vi "ABB Test Cooling curve.vi"(10 "Measure":enum16{"Full Load", "Partial Load", "No Load"}(ring), 11 "Heat run Type":enum16{"Full Load", "Partial- & No-Load"}(ring)) -> ()   [LabVIEW 2017]
uses:
  ABB global.vi
panel:
  in  "Slip Ring Temperatures (° C)":cluster{"K":dbl, "L":dbl, "M ":dbl}
  out "Selection":T1 {"Rotor dT" format="%#.2g"; "Rotor R" format="%#.6g"; "Stator dT" format="%#.2g"; "Stator R" format="%#.6g"}
  in  "Use":bool
  out "Rotor Fitted Zero time  R":dbl format="%.4f"
  out "Type of Run":string
  in  "Stop":bool
  out "Elapsed time (secs)":dbl format="%#.1f"
  in  "Start":bool
  in  "Enter Rotor Res.":dbl
  in  "Enter Stator Res.":dbl
  in  "Select Resistance":T2(ring)
  out "Motor Type":string
  out "Cooling in Temp (°C)":dbl
  out "error":dbl
  in  "y":dbl step=0.01
  out "Stator Fitted Zero time  R":dbl format="%.4f"
  out "Selected Entries 2":string[](array[string])
  out "Cold resistance":T3 {"Temperature(°C)" format="%#.2g"}
  in  "Rotor Cooling Curve Data":string[][](table)
  out "Rotor":cluster{dbl[], dbl[]}[](graph)
  out "Rotor Readings":string[][](table)
  in  "Stator Cooling Curve Data":string[][](table)
  out "Stator":cluster{dbl[], dbl[]}[](graph)
  out "Stator Readings":string[][](table)
  out "Serial number":string
  out "W.O number":string
  out "Timedate":string
  in  "Exit":bool
  # "?"
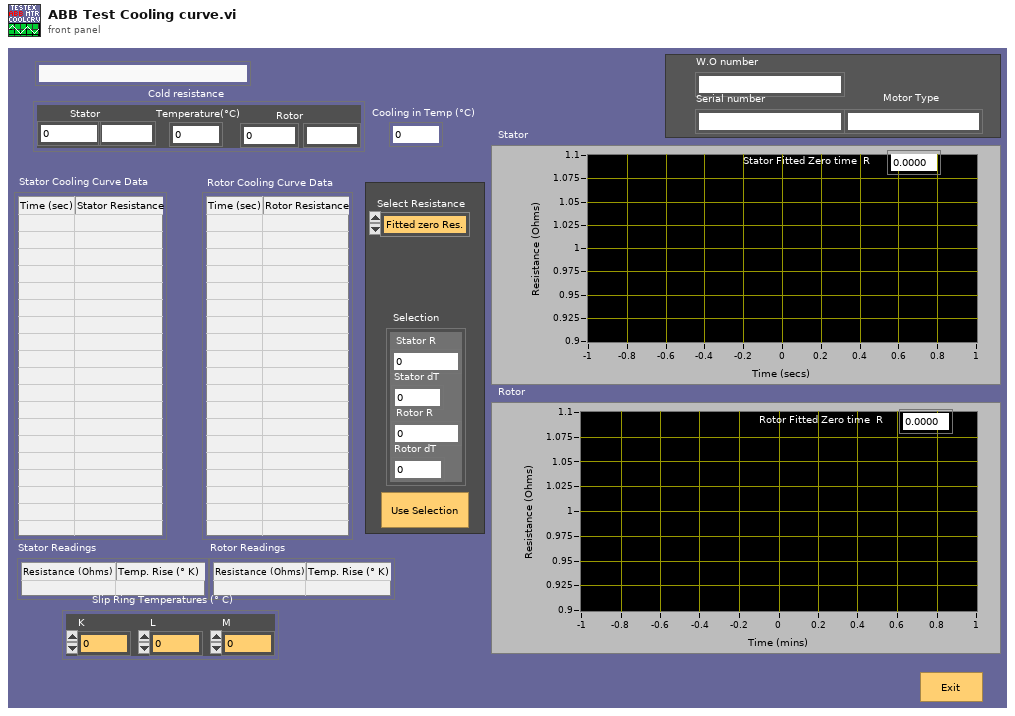
[diagram p1: front panel]
types:
  T1 = cluster{"Stator R":dbl, "Stator dT":dbl, "Rotor R":dbl, "Rotor dT":dbl}
  T2 = enum16{"Fitted zero Res.", "Selected Res.", "Entered Res."}
  T3 = cluster{"Stator":dbl, "Rotor":dbl, "Stator Units":string, "Rotor Units":string, "Temperature(°C)":dbl}
  T4 = cluster{"Stator R":dbl, "Stator dT":dbl, "Rotor R":dbl, "Rotor dT":dbl, "Stator Cooling curve":dbl[][], "Rotor Cooling curve":dbl[][], "Select Resistance":enum16{"Fitted zero Res.", "Selected Res.", "Entered Res."}}[]
  T5 = cluster{"Stator R":dbl, "Stator dT":dbl, "Rotor R":dbl, "Rotor dT":dbl, "Stator Cooling curve":dbl[][], "Rotor Cooling curve":dbl[][], "Select Resistance":enum16{"Fitted zero Res.", "Selected Res.", "Entered Res."}}
  T6 = cluster{"Simulate Norma":bool, "Norma 5000 Address":u8, "WebDaq IP Address":string, "Simulate cDAQ":bool}
  T7 = typedef "LVRowAndColumnTypeDef.ctl" = cluster{"Row":i32, "Column":i32}
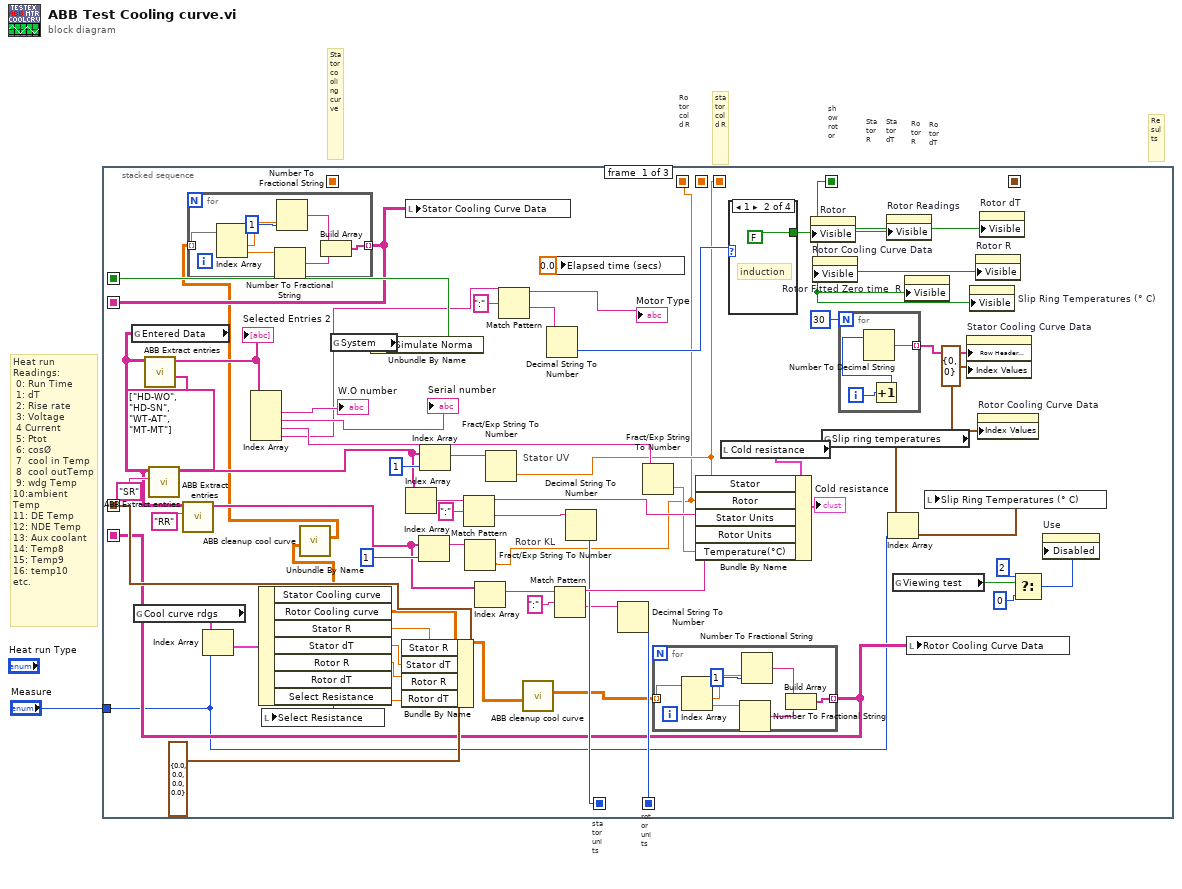
[diagram p0: block diagram]
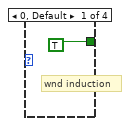
[diagram p2: hidden frame]
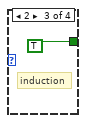
[diagram p3: hidden frame]
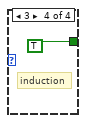
[diagram p4: hidden frame]
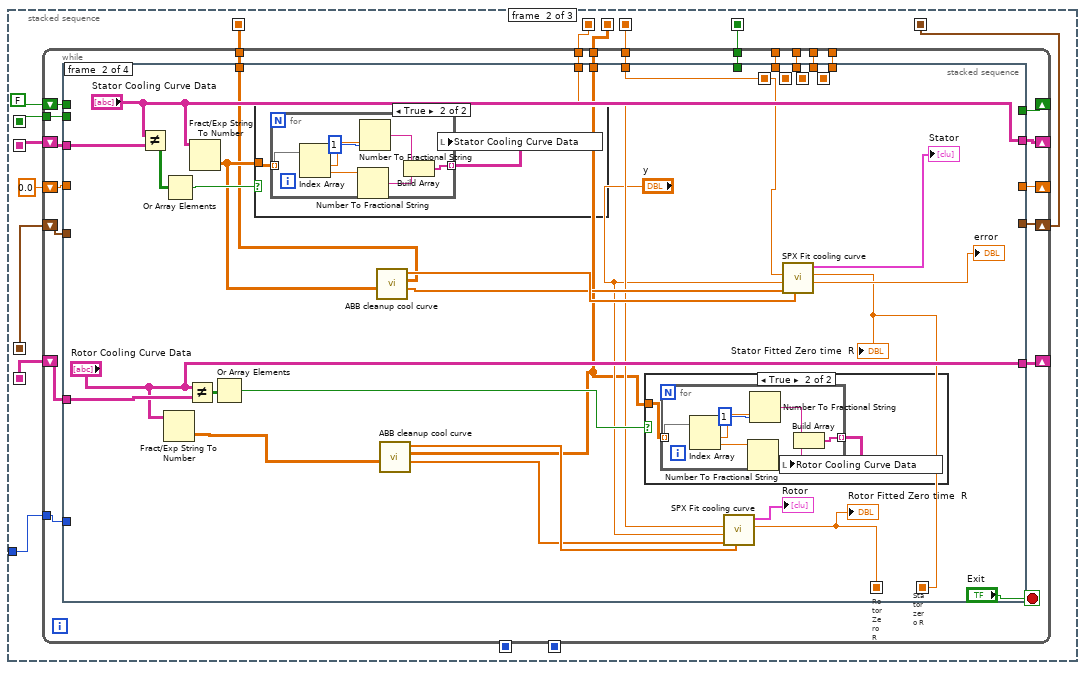
[diagram p5: hidden frame]
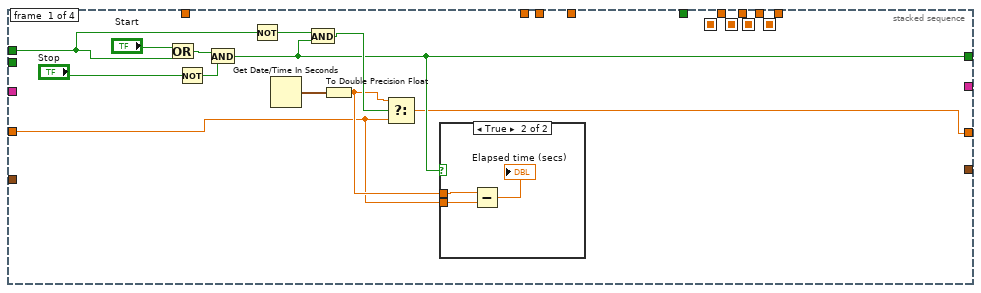
[diagram p6: hidden frame]
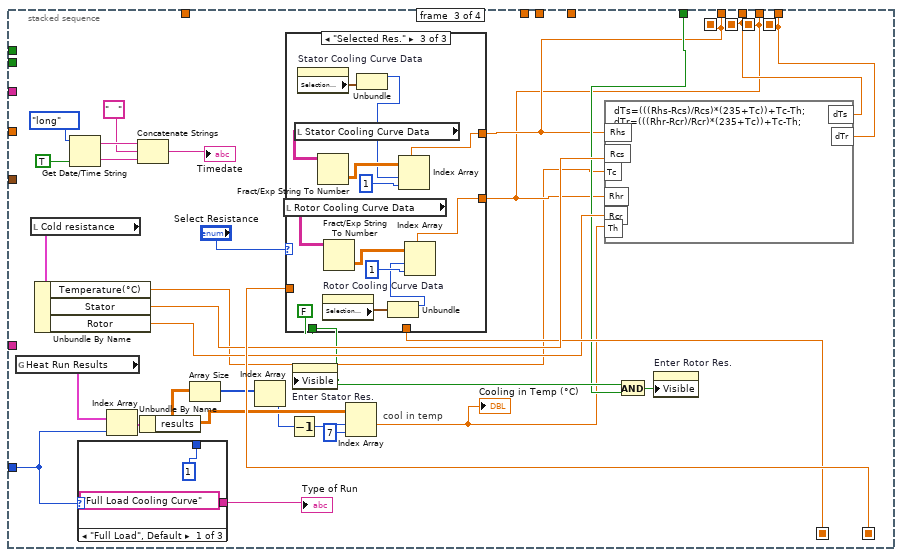
[diagram p10: hidden frame]
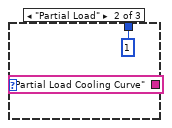
[diagram p11: hidden frame]
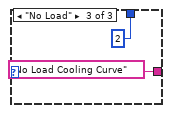
[diagram p12: hidden frame]
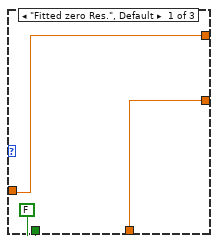
[diagram p13: hidden frame]
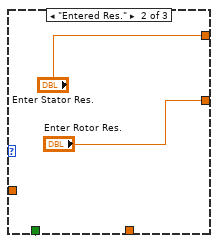
[diagram p14: hidden frame]
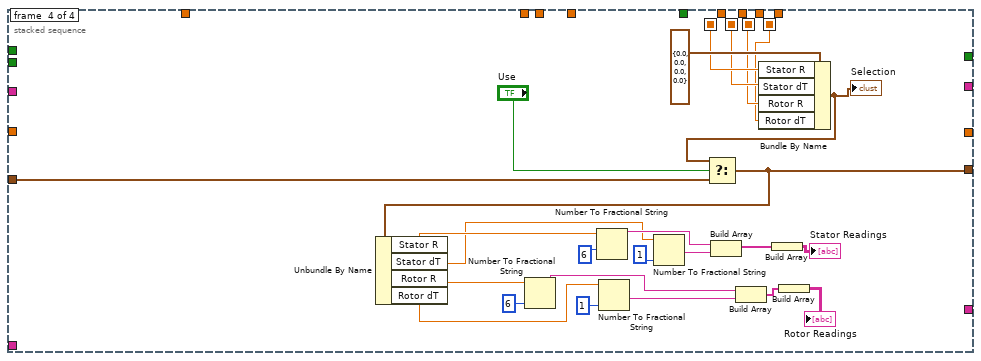
[diagram p15: hidden frame]
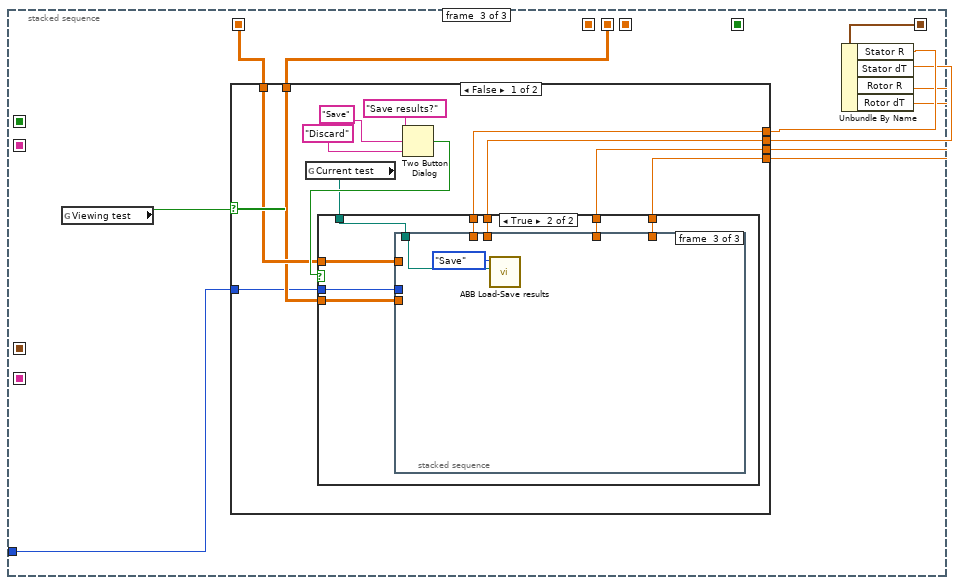
[diagram p16: hidden frame]
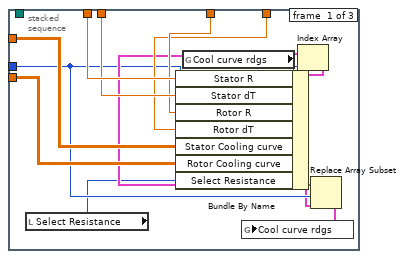
[diagram p18: hidden frame]
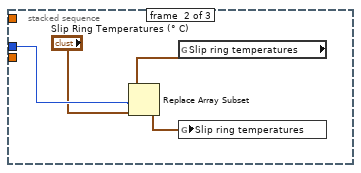
[diagram p19: hidden frame]
diagram:
  # "StatordT"
  # "RotordT"
  # "Rotor R"
  # "Stator R"
  # "show rotor"
  # "Rotor cold R"
  # "Heat run Readings:\n 0: Run Time\n 1: dT\n 2: Rise rate\n 3: Voltage\n 4 Current\n 5: Ptot\n 6: cosØ\n 7  cool in Temp\n 8  cool outTemp\n 9: wdg Temp\n10:ambient Temp\n11: DE Temp\n12: NDE Temp\n13: Aux coolant\n14: Temp8\n15: Temp9\n16: temp10\netc."
  # "rotor units"
  # "stator units"
  # "Stator cooling curve"
  # "stator cold R"
  # "Results"
  n1 = stacked-sequence {
    seq-local: [w63 _ _] -> [_ w98 _]
    seq-local: [w10 _ _] -> [_ w97 _]
    seq-local: [_ w96 _] -> [_ _ w265]
    seq-local: [_ w95 _] -> [_ _ w264]
    seq-local: [w11 _ _] -> [_ w94 _]
    seq-local: [w19 _ _] -> [_ w93 _]
    seq-local: [w32 _ _] -> [_ _ _]
    seq-local: [w30 _ _] -> [_ _ _]
    seq-local: [w18 _ _] -> [_ w92 _]
    seq-local: [w8 _ _] -> [_ w91 _]
    seq-local: [w20 _ _] -> [_ w87 _]
    seq-local: [_ w86 _] -> [_ _ w262]
    tunnel: "Measure" -> [w2 w88 w263]
    frame #0 {
      w5 = cluster{"Row":i32, "Column":i32} {"Row"=0, "Column"=0} ("Edit Position")
      # "Rotor KL"
      # "Stator UV"
      n2 = global read "ABB global.vi" "Entered Data"() -> (w56:string[][])
      n3 = global read "ABB global.vi" "Cool curve rdgs"() -> (w27:T4)
      n4 = call "ABB Extract entries.vi"("Entry IDs"=string[] ["HD-WO", "HD-SN", "WT-AT", "MT-MT"], "Entry table in"=w56) -> ("Selected Entries"=w39:string[])  [unwired: 9 in]
      "Selected Entries 2" <- w39
      n5 = call "ABB Extract entries.vi"("Entry ID"="SR", "Entry table in"=w56) -> ("Selected Entries"=w50:string[])  [unwired: 9 in]
      n6 = call "ABB Extract entries.vi"("Entry ID"="RR", "Entry table in"=w56) -> ("Selected Entries"=w43:string[])  [unwired: 9 in]
      n7 = Index Array(array=w27, index=w2) -> (element=w26:T5)
      n8 = Index Array(array=w39) -> (element #1=→"W.O number":string, element #2=→"Serial number":string, element #3=w40:string, element #4=w35:string)  [unwired: 4 in]
      n9 = Unbundle By Name(w26) -> ("Stator Cooling curve"=w12:dbl[][], "Rotor Cooling curve"=w9:dbl[][], "Stator R"=w25:dbl, "Stator dT"=w24:dbl, "Rotor R"=w23:dbl, "Rotor dT"=w22:dbl, "Select Resistance"=w13:T2)
      n10 = local write "Select Resistance"(w13) -> ()
      n11 = call "ABB cleanup cool curve.vi"("cool curve in"=w12) -> ("Cool curve out"=w7:dbl[][])  [unwired: 8 in, 2 out]
      n12 = for {
        tunnel: w7 -> [w78] mode=indexing
        tunnel: [w74] -> w11 mode=indexing
        n13 = Index Array(array=w78) -> (element #1=w76:dbl, element #2=w75:dbl)  [unwired: 2 in]
        n14 = Number To Fractional String(number=w75) -> (F-format string=w73:string)  [unwired: 3 in]
        n15 = Number To Fractional String(number=w76, precision (6)=i16 1) -> (F-format string=w72:string)  [unwired: 2 in]
        n16 = Build Array(w72, w73) -> (w74:string[])
      }
      n17 = global read "ABB global.vi" "System"() -> (w64:T6)
      n18 = Unbundle By Name(w64) -> ("Simulate Norma"=w63:bool)
      n19 = Bundle By Name(cluster=T1 {"Stator R"=0.0, "Stator dT"=0.0, "Rotor R"=0.0, "Rotor dT"=0.0} ("Selection"), "Stator R"=w25, "Stator dT"=w24, "Rotor R"=w23, "Rotor dT"=w22) -> (w20:T1)
      n20 = local write "Stator Cooling Curve Data"(w11) -> ()
      n21 = Index Array(array=w50) -> (element=w49:string)  [unwired: 1 in]
      n22 = Index Array(array=w43, index=1) -> (element=w45:string)
      n23 = Index Array(array=w50, index=1) -> (element=w53:string)
      n24 = Match Pattern(string=w49, regular expression=":") -> (before substring=w42:string, after substring=w33:string)  [unwired: 1 in, 2 out]
      n25 = Fract/Exp String To Number(string=w45) -> (number=w18:dbl)  [unwired: 3 in, 1 out]
      n26 = Index Array(array=w43) -> (element=w46:string)  [unwired: 1 in]
      n27 = Fract/Exp String To Number(string=w53) -> (number=w19:dbl)  [unwired: 3 in, 1 out]
      n28 = Match Pattern(string=w35, regular expression=":") -> (before substring=→"Motor Type":string, after substring=w37:string)  [unwired: 1 in, 2 out]
      n29 = call "ABB cleanup cool curve.vi"("cool curve in"=w9) -> ("Cool curve out"=w6:dbl[][])  [unwired: 8 in, 2 out]
      n30 = Decimal String To Number(string=w37) -> (number=w34:i32)  [unwired: 2 in, 1 out]
      n31 = local write "Elapsed time (secs)"(0.0 ("Elapsed time (secs)")) -> ()
      n32 = Match Pattern(string=w46, regular expression=":") -> (before substring=w41:string, after substring=w31:string)  [unwired: 1 in, 2 out]
      n33 = Decimal String To Number(string=w33) -> (number=w32:i32)  [unwired: 2 in, 1 out]
      n34 = Decimal String To Number(string=w31) -> (number=w30:i32)  [unwired: 2 in, 1 out]
      n35 = Fract/Exp String To Number(string=w40) -> (number=w29:dbl)  [unwired: 3 in, 1 out]
      n36 = for {
        tunnel: w6 -> [w71] mode=indexing
        tunnel: [w67] -> w10 mode=indexing
        n37 = Index Array(array=w71) -> (element #1=w69:dbl, element #2=w68:dbl)  [unwired: 2 in]
        n38 = Number To Fractional String(number=w68) -> (F-format string=w66:string)  [unwired: 3 in]
        n39 = Number To Fractional String(number=w69, precision (6)=i16 1) -> (F-format string=w65:string)  [unwired: 2 in]
        n40 = Build Array(w65, w66) -> (w67:string[])
      }
      n41 = local read "Cold resistance"() -> (w52:T3)
      n42 = Bundle By Name(cluster=w52, "Stator"=w19, "Rotor"=w18, "Stator Units"=w42, "Rotor Units"=w41, "Temperature(°C)"=w29) -> (→"Cold resistance":T3)
      n43 = case shown="1" w34 {
        tunnel: [TRUE FALSE TRUE TRUE] -> w8
        frame 0, Default {
          # "wnd induction"
        }
        frame 1 {
          # "induction"
        }
        frame 2 {
          # "induction"
        }
        frame 3 {
          # "induction"
        }
      }
      n44 = property on="Rotor" class="XYGraph (strict)"("Visible"=w8) -> ()  [unwired: 2 in, 2 out]
      n45 = property on="Rotor Cooling Curve Data" class="Tbl (strict)"("Visible"=w8) -> ()  [unwired: 2 in, 2 out]
      n46 = global read "ABB global.vi" "Slip ring temperatures"() -> (w4:cluster{"K":dbl, "L":dbl, "M ":dbl}[])
      n47 = for {
        N: 30 -> [_]
        tunnel: [w83] -> w61 mode=indexing
        i -> [w85]
        n48 = Increment(x=w85) -> (x+1=w84:i32)
        n49 = Number To Decimal String(number=w84) -> (decimal integer string=w83:string)  [unwired: 1 in]
      }
      n50 = property on="Rotor Readings" class="Tbl (strict)"("Visible"=w8) -> ()  [unwired: 2 in, 2 out]
      n51 = Index Array(array=w4, index=w2) -> (element=w3:cluster{"K":dbl, "L":dbl, "M ":dbl})
      n52 = global read "ABB global.vi" "Viewing test"() -> (w17:bool)
      n53 = property on="Rotor Fitted Zero time  R" class="DigNum (strict)"("Visible"=w8) -> ()  [unwired: 2 in, 2 out]
      n54 = local write "Rotor Cooling Curve Data"(w10) -> ()
      n55 = local write "Slip Ring Temperatures (° C)"(w3) -> ()
      n56 = property on="Stator Cooling Curve Data" class="Tbl (strict)"("Row Header Strings[]"=w61, "Index Values"=w5) -> ()  [unwired: 2 in, 2 out]
      n57 = property on="Slip Ring Temperatures (° C)" class="Clust (strict)"("Visible"=w8) -> ()  [unwired: 2 in, 2 out]
      n58 = property on="Rotor R" class="DigNum (strict)"("Visible"=w8) -> ()  [unwired: 2 in, 2 out]
      n59 = property on="Rotor Cooling Curve Data" class="Tbl (strict)"("Index Values"=w5) -> ()  [unwired: 2 in, 2 out]
      n60 = property on="Rotor dT" class="DigNum (strict)"("Visible"=w8) -> ()  [unwired: 2 in, 2 out]
      n61 = Select(t=2, s=w17, f=0) -> (s? t:f=w14:i32)
      n62 = property on="Use" class="Bool"("Disabled"=w14) -> ()  [unwired: 2 in, 2 out]
    }
    frame #1 {
      # "Stator zero R"
      n63 = while {
        tunnel: w98 -> [w119]
        shift-right: [w117] -> _
        shift-left: w94 -> [w118]
        shift-right: [w116] -> _
        shift-left: w97 -> [w115]
        tunnel: [w114] -> w96
        tunnel: [w113] -> w95
        tunnel: w93 -> [w112]
        tunnel: w92 -> [w111]
        tunnel: w91 -> [w110]
        shift-right: [w106] -> _
        shift-left: 0.0 -> [w109]
        shift-right: [w107] -> _
        shift-left: FALSE -> [w108]
        tunnel: [w105] -> _
        tunnel: [w104] -> _
        tunnel: [w103] -> _
        tunnel: [w102] -> _
        tunnel: w88 -> [w101]
        shift-right: [w100] -> w86
        shift-left: w87 -> [w99]
        stop <- "Exit" stop-if-true
        # "Rotor Zero R"
        n64 = stacked-sequence {
          seq-local: [_ w145 _ _] -> [_ _ w200 _]
          seq-local: [_ w141 _ _] -> [_ _ w190 _]
          seq-local: [_ _ w183 _] -> [_ _ _ w256]
          seq-local: [_ _ w182 _] -> [_ _ _ w255]
          seq-local: [_ _ w181 _] -> [_ _ _ w254]
          seq-local: [_ _ w180 _] -> [_ _ _ w253]
          tunnel: w119 -> [_ _ _ _]
          tunnel: w118 -> [_ w159 _ _]
          tunnel: [_ "Stator Cooling Curve Data" _ _] -> w117
          tunnel: [_ "Rotor Cooling Curve Data" _ _] -> w116
          tunnel: w115 -> [_ w155 _ _]
          tunnel: [_ w137 _ _] -> w114
          tunnel: [_ w136 _ _] -> w113
          tunnel: w112 -> [_ w150 _ _]
          tunnel: w111 -> [_ w144 _ _]
          tunnel: w110 -> [_ _ w186 _]
          tunnel: w109 -> [w121 _ _ _]
          tunnel: w108 -> [w126 _ _ _]
          tunnel: [w124 _ _ _] -> w107
          tunnel: [w122 _ _ _] -> w106
          tunnel: [_ _ w183 _] -> w105
          tunnel: [_ _ w182 _] -> w104
          tunnel: [_ _ w180 _] -> w103
          tunnel: [_ _ w181 _] -> w102
          tunnel: w101 -> [_ _ w185 _]
          tunnel: [_ _ _ w239] -> w100
          tunnel: w99 -> [_ _ _ w250]
          frame #0 {
            n65 = Or(x="Start", y=w126) -> (x .or. y?=w130:bool)
            n66 = Not(x="Stop") -> (.not. x?=w129:bool)
            n67 = And(x=w130, y=w129) -> (x .and. y?=w124:bool)
            n68 = Not(x=w126) -> (.not. x?=w127:bool)
            n69 = Get Date/Time In Seconds() -> (seconds since 1Jan1904=w132:timestamp)
            n70 = And(x=w127, y=w124) -> (x .and. y?=w125:bool)
            n71 = To Double Precision Float(number=w132) -> (double precision float=w123:dbl)
            n72 = Select(t=w123, s=w125, f=w121) -> (s? t:f=w122:dbl)
            n73 = case shown="True" w124 {
              tunnel: w123 -> [_ w135]
              tunnel: w121 -> [_ w134]
              frame False {
              }
              frame True {
                n74 = Subtract(x=w135, y=w134) -> (x-y=→"Elapsed time (secs)":dbl)
              }
            }
          }
          frame #1 {
            n75 = Not Equal?(x="Stator Cooling Curve Data", y=w159) -> (x != y?=w158:bool[][])
            n76 = Fract/Exp String To Number(string="Rotor Cooling Curve Data") -> (number=w140:dbl[][])  [unwired: 3 in, 1 out]
            n77 = Or Array Elements(Boolean array=w158) -> (logical OR=w157:bool)
            n78 = Not Equal?(x="Rotor Cooling Curve Data", y=w155) -> (x != y?=w154:bool[][])
            n79 = Fract/Exp String To Number(string="Stator Cooling Curve Data") -> (number=w151:dbl[][])  [unwired: 3 in, 1 out]
            n80 = Or Array Elements(Boolean array=w154) -> (logical OR=w152:bool)
            n81 = case shown="True" w157 {
              tunnel: w151 -> [_ w170]
              frame False {
              }
              frame True {
                n82 = for {
                  tunnel: w170 -> [w177] mode=indexing
                  tunnel: [w173] -> w169 mode=indexing
                  n83 = Index Array(array=w177) -> (element #1=w175:dbl, element #2=w174:dbl)  [unwired: 2 in]
                  n84 = Number To Fractional String(number=w174) -> (F-format string=w172:string)  [unwired: 3 in]
                  n85 = Number To Fractional String(number=w175, precision (6)=i16 1) -> (F-format string=w171:string)  [unwired: 2 in]
                  n86 = Build Array(w171, w172) -> (w173:string[])
                }
                n87 = local write "Stator Cooling Curve Data"(w169) -> ()
              }
            }
            n88 = call "ABB cleanup cool curve.vi"("cool curve in"=w151) -> ("Time"=w148:dbl[], "Cool curve out"=w137:dbl[][], "Resistance"=w149:dbl[])  [unwired: 8 in]
            n89 = call "ABB cleanup cool curve.vi"("cool curve in"=w140) -> ("Time"=w138:dbl[], "Cool curve out"=w136:dbl[][], "Resistance"=w139:dbl[])  [unwired: 8 in]
            n90 = case shown="True" w152 {
              tunnel: w136 -> [_ w161]
              frame False {
              }
              frame True {
                n91 = for {
                  tunnel: w161 -> [w168] mode=indexing
                  tunnel: [w164] -> w160 mode=indexing
                  n92 = Index Array(array=w168) -> (element #1=w166:dbl, element #2=w165:dbl)  [unwired: 2 in]
                  n93 = Number To Fractional String(number=w165) -> (F-format string=w163:string)  [unwired: 3 in]
                  n94 = Number To Fractional String(number=w166, precision (6)=i16 1) -> (F-format string=w162:string)  [unwired: 2 in]
                  n95 = Build Array(w162, w163) -> (w164:string[])
                }
                n96 = local write "Rotor Cooling Curve Data"(w160) -> ()
              }
            }
            n97 = call "SPX Fit cooling curve.vi"("Resistances"=w139, "Time"=w138, "Radj"="y", "cold R"=w144) -> ("Zero R"=w141:dbl, "Stator"=→"Rotor":cluster{dbl[], dbl[]}[])  [unwired: 5 in, 1 out]
            "Rotor Fitted Zero time  R" <- w141
            n98 = call "SPX Fit cooling curve.vi"("Resistances"=w149, "Time"=w148, "Radj"="y", "cold R"=w150) -> ("error"=→"error":dbl, "Zero R"=w145:dbl, "Stator"=→"Stator":cluster{dbl[], dbl[]}[])  [unwired: 5 in]
            "Stator Fitted Zero time  R" <- w145
          }
          frame #2 {
            # "cool in temp"
            n99 = global read "ABB global.vi" "Heat Run Results"() -> (w197:cluster{"results":dbl[][], "Comments":string}[])
            n100 = local read "Cold resistance"() -> (w199:T3)
            n101 = Unbundle By Name(w199) -> ("Temperature(°C)"=w179:dbl, "Stator"=w198:dbl, "Rotor"=w189:dbl)
            n102 = Get Date/Time String(date format (0)=enum16{"short", "long", "abbreviated"}."long", want seconds? (F)=TRUE) -> (date string=w205:string, time string=w204:string)  [unwired: 1 in]
            n103 = case shown="\"Full Load\", Default" w185 {
              tunnel: ["Full Load Cooling Curve" "Partial Load Cooling Curve" "No Load Cooling Curve"] -> w184
              tunnel: [1 1 2] -> _
              frame "Full Load", Default {
              }
              frame "Partial Load" {
              }
              frame "No Load" {
              }
            }
            "Type of Run" <- w184
            n104 = Index Array(array=w197, index=w185) -> (element=w196:cluster{"results":dbl[][], "Comments":string})
            n105 = Concatenate Strings(w205, "   ", w204) -> (→"Timedate":string)
            n106 = Unbundle By Name(w196) -> ("results"=w194:dbl[][])
            n107 = Array Size(array=w194) -> (size(s)=w195:i32[])
            n108 = Index Array(array=w195) -> (element=w193:i32)  [unwired: 1 in]
            n109 = case shown="\"Selected Res.\"" "Select Resistance" {
              tunnel: w200 -> [w215 _ _]
              tunnel: [FALSE TRUE FALSE] -> w188
              tunnel: [w215 "Enter Stator Res." w228] -> w183
              tunnel: [w214 "Enter Rotor Res." w222] -> w181
              tunnel: w190 -> [w214 _ _]
              frame "Fitted zero Res.", Default {
              }
              frame "Entered Res." {
              }
              frame "Selected Res." {
                n110 = local read "Rotor Cooling Curve Data"() -> (w223:string[][])
                n111 = local read "Stator Cooling Curve Data"() -> (w231:string[][])
                n112 = property on="Stator Cooling Curve Data" class="Tbl (strict)"() -> ("Selection Start"=w227:T7)  [unwired: 2 in, 2 out]
                n113 = Fract/Exp String To Number(string=w231) -> (number=w230:dbl[][])  [unwired: 3 in, 1 out]
                n114 = property on="Rotor Cooling Curve Data" class="Tbl (strict)"() -> ("Selection Start"=w221:T7)  [unwired: 2 in, 2 out]
                n115 = Fract/Exp String To Number(string=w223) -> (number=w224:dbl[][])  [unwired: 3 in, 1 out]
                n116 = Unbundle(w227) -> ("Row"=w226:i32)  [unwired: 1 out]
                n117 = Unbundle(w221) -> ("Row"=w220:i32)  [unwired: 1 out]
                n118 = Index Array(array=w230, index (row)=w226, index (col)=1 ("disabled index (col)")) -> (element=w228:dbl)
                n119 = Index Array(array=w224, index (row)=w220, index (col)=1 ("disabled index (col)")) -> (element=w222:dbl)
              }
            }
            n120 = Decrement(x=w193) -> (x-1=w192:i32)
            n121 = property on="Enter Stator Res." class="DigNum (strict)"("Visible"=w188) -> ()  [unwired: 2 in, 2 out]
            n122 = Index Array(array=w194, index (row)=w192, index (col)=7 ("disabled index (col)")) -> (element=w178:dbl)
            "Cooling in Temp (°C)" <- w178
            n123 = formula code="dTs=(((Rhs-Rcs)/Rcs)*(235+Tc))+Tc-Th;\ndTr=(((Rhr-Rcr)/Rcr)*(235+Tc))+Tc-Th;"("Rhs"=w183, "Rcs"=w198, "Tc"=w179, "Rhr"=w181, "Rcr"=w189, "Th"=w178) -> ("dTs"=w182:dbl, "dTr"=w180:dbl)
            n124 = And(x=w188, y=w186) -> (x .and. y?=w187:bool)
            n125 = property on="Enter Rotor Res." class="DigNum (strict)"("Visible"=w187) -> ()  [unwired: 2 in, 2 out]
          }
          frame #3 {
            n126 = Bundle By Name(cluster=T1 {"Stator R"=0.0, "Stator dT"=0.0, "Rotor R"=0.0, "Rotor dT"=0.0} ("Selection"), "Stator R"=w256, "Stator dT"=w255, "Rotor R"=w254, "Rotor dT"=w253) -> (w251:T1)
            "Selection" <- w251
            n127 = Select(t=w251, s="Use", f=w250) -> (s? t:f=w239:T1)
            n128 = Unbundle By Name(w239) -> ("Stator R"=w238:dbl, "Stator dT"=w237:dbl, "Rotor R"=w236:dbl, "Rotor dT"=w235:dbl)
            n129 = Number To Fractional String(number=w236, precision (6)=i16 6) -> (F-format string=w243:string)  [unwired: 2 in]
            n130 = Number To Fractional String(number=w238, precision (6)=i16 6) -> (F-format string=w246:string)  [unwired: 2 in]
            n131 = Number To Fractional String(number=w235, precision (6)=i16 1) -> (F-format string=w242:string)  [unwired: 2 in]
            n132 = Number To Fractional String(number=w237, precision (6)=i16 1) -> (F-format string=w248:string)  [unwired: 2 in]
            n133 = Build Array(w246, w248) -> (w245:string[])
            n134 = Build Array(w243, w242) -> (w240:string[])
            n135 = Build Array(w245) -> (→"Stator Readings":string[][])
            n136 = Build Array(w240) -> (→"Rotor Readings":string[][])
          }
        }
      }
    }
    frame #2 {
      n137 = global read "ABB global.vi" "Viewing test"() -> (w266:bool)
      n138 = Unbundle By Name(w262) -> ("Stator R"=w261:dbl, "Stator dT"=w260:dbl, "Rotor R"=w259:dbl, "Rotor dT"=w258:dbl)
      n139 = case shown="False" w266 {
        tunnel: w265 -> [w276 _]
        tunnel: w264 -> [w274 _]
        tunnel: w261 -> [w273 _]
        tunnel: w260 -> [w272 _]
        tunnel: w259 -> [w271 _]
        tunnel: w258 -> [w270 _]
        tunnel: w263 -> [w267 _]
        frame False {
          n140 = global read "ABB global.vi" "Current test"() -> (w275:path)
          n141 = Two Button Dialog(message="Save results?", 1:"Discard" ("F button name (\"Cancel\")"), 2:"Save" ("T button name (\"OK\")")) -> (T button?=w277:bool)
          n142 = case shown="True" w277 {
            tunnel: w276 -> [_ w285]
            tunnel: w275 -> [_ w286]
            tunnel: w274 -> [_ w284]
            tunnel: w273 -> [_ w283]
            tunnel: w272 -> [_ w282]
            tunnel: w271 -> [_ w281]
            tunnel: w270 -> [_ w280]
            tunnel: w267 -> [_ w279]
            frame False {
            }
            frame True {
              n143 = stacked-sequence {
                tunnel: w286 -> [_ _ w303]
                tunnel: w285 -> [w297 _ _]
                tunnel: w284 -> [w298 _ _]
                tunnel: w283 -> [w296 _ _]
                tunnel: w282 -> [w295 _ _]
                tunnel: w281 -> [w294 _ _]
                tunnel: w280 -> [w293 _ _]
                tunnel: w279 -> [w290 w302 _]
                frame #0 {
                  n144 = local read "Select Resistance"() -> (w287:T2)
                  n145 = global read "ABB global.vi" "Cool curve rdgs"() -> (w291:T4)
                  n146 = Index Array(array=w291, index=w290) -> (element=w292:T5)
                  n147 = Bundle By Name(cluster=w292, "Stator R"=w296, "Stator dT"=w295, "Rotor R"=w294, "Rotor dT"=w293, "Stator Cooling curve"=w297, "Rotor Cooling curve"=w298, "Select Resistance"=w287) -> (w288:T5)
                  n148 = Replace Array Subset(array=w291, new element=w288, index=w290) -> (w289:T4)
                  n149 = global write "ABB global.vi" "Cool curve rdgs"(w289) -> ()
                }
                frame #1 {
                  n150 = global read "ABB global.vi" "Slip ring temperatures"() -> (w301:cluster{"K":dbl, "L":dbl, "M ":dbl}[])
                  n151 = Replace Array Subset(array=w301, new element="Slip Ring Temperatures (° C)", index=w302) -> (w300:cluster{"K":dbl, "L":dbl, "M ":dbl}[])
                  n152 = global write "ABB global.vi" "Slip ring temperatures"(w300) -> ()
                }
                frame #2 {
                  n153 = call "ABB Load-Save results.vi"("Path"=w303, "Mode"=enum16{"LOAD", "Save"}."Save") -> ()  [unwired: 10 in]
                }
              }
            }
          }
        }
        frame True {
        }
      }
    }
  }
